vi "_setOtherRef.vi"(7 "parentURL":string, 8 "error in (no error)":errorcluster, 9 "Name":string, 10 "Refnum":variant, 11 "TagDB in":T1) -> (0 "error out":errorcluster, 2 "Ref-Key":string, 3 "TagDB out":T1)   [LabVIEW 2014, in "RefManager(dev).lvlib"]
uses:
  RefManager(dev).lvlib
  <userlib>/_NEVSTOP/TagDB/Core/tagDB_Def.ctl
  <userlib>/_NEVSTOP/TagDB/Core/_Support/Access/_setAnything.vi
  <userlib>/_NEVSTOP/TagDB/Core/_XNode/tagDB_setValue.xnode/tagDB_setValue.xnode
  <userlib>/_NEVSTOP/TagDB/Core/TagDB.lvlib
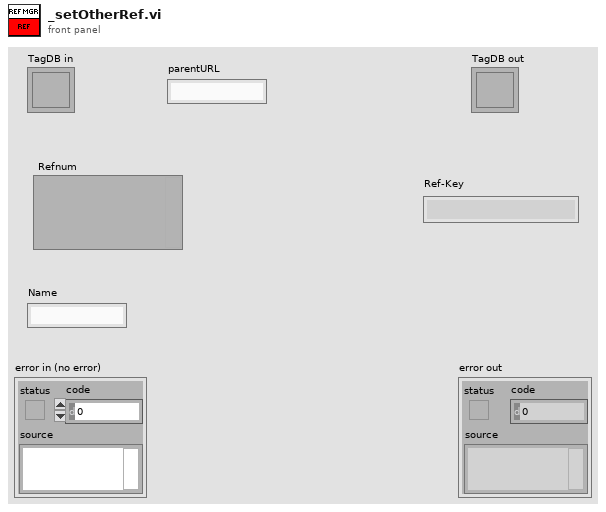
[diagram p1: front panel]
types:
  T1 = typedef "TagDB.lvlib/tagDB_Def.ctl" = refnum<k1>
  T2 = enum8{"Generic", "Datalog File Refnum", "Byte Stream File Refnum", "Device Refnum", "Occurence Refnum", "TCP Connection Refnum", "VISA Refnum (Obsolete)", "Automation Renum", "VI Server Refnum", "Menu Refnum", "IVI Refnum (Obsolete)", "IMAQ Session", "0x0C", "Datasocket Refnum", "VISA Resource", "IVI Logical Name", "UDP Connection Refnum", "Notifier Refnum", "Queue Refnum", "IrDA Refnum", "Hardware Plugin Refnum", "Hardware Plugin Tag Refnum", "DAQmx Refnum", "Event Registration Refnum", ".NET Refnum", "User Event Refnum", "0x1A", "Event Callback", "0x1C", "0x1D", "Only Used Internal to LabVIEW", "Bluetooth", "Data Value References", "RT FIFO", "TDM Streaming"}
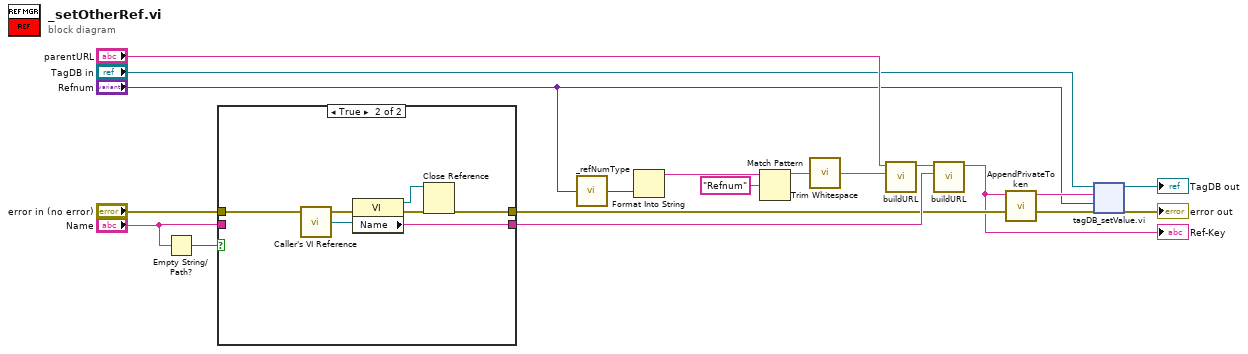
[diagram p0: block diagram]
diagram:
  n1 = Empty String/Path?(string/path="Name") -> (empty?=w18:bool)
  n2 = case shown="True" w18 {
    tunnel: [w20 w21] -> w9
    tunnel: "Name" -> [w20 _]
    tunnel: "error in (no error)" -> [w19 w23]
    tunnel: [w19 w22] -> w3
    frame False {
    }
    frame True {
      n3 = call "Caller's VI Reference.vi"("error in (no error)"=w23) -> ("error out"=w27:errorcluster, "Caller's VI Reference"=w26:refnum<vi>)  [unwired: 5 in]
      n4 = property on="Property Node" class="VI"(reference=w26, error in=w27) -> (reference out=w25:refnum<vi>, error out=w24:errorcluster, "Name"=w21:string)
      n5 = Close Reference(reference=w25, error in (no error)=w24) -> (error out=w22:errorcluster)
    }
  }
  n6 = call <userlib>:"_refNumType.vi"("Data"="Refnum") -> ("Refnum Subtype Enum"=w14:T2)  [unwired: 4 in]
  n7 = Format Into String(w14) -> (resulting string=w12:string)  [unwired: 3 in, 1 out]
  n8 = Match Pattern(string=w12, regular expression="Refnum") -> (before substring=w10:string)  [unwired: 1 in, 3 out]
  n9 = call <vilib>:"Trim Whitespace.vi"("string"=w10) -> ("trimmed string"=w13:string)  [unwired: 1 in]
  n10 = call <userlib>:"buildURL.vi"("DataName"=w13, "parentURL"="parentURL") -> ("DataURL"=w15:string)  [unwired: 9 in]
  n11 = call <userlib>:"buildURL.vi"("DataName"=w9, "parentURL"=w15) -> ("DataURL"=w1:string)  [unwired: 9 in]
  "Ref-Key" <- w1
  n12 = call <userlib>:"AppendPrivateToken.vi"("DataURL"=w1) -> ("String"=w5:string)  [unwired: 10 in]
  n13 = xnode "tagDB_setValue.vi"("DB Ref"="TagDB in", "name"=w5, "value"="Refnum", "Error In"=w3) -> ("DB Ref(dup)"=→"TagDB out":T1, "Error Out"=→"error out":errorcluster)  [unwired: 1 out]
